vi "强度图.vi"() -> ()   [LabVIEW 2020]
doc: "本VI是为《我和LabVIEW》一书编写的示例。\n关于本书的介绍请参考网页：\nhttp://ruanqizhen.spaces.live.com/blog/cns!5852D4F797C53FB6!4310.entry"
panel:
  out "表格控件":string[][](table)
  out "强度图":dbl[][](graph)
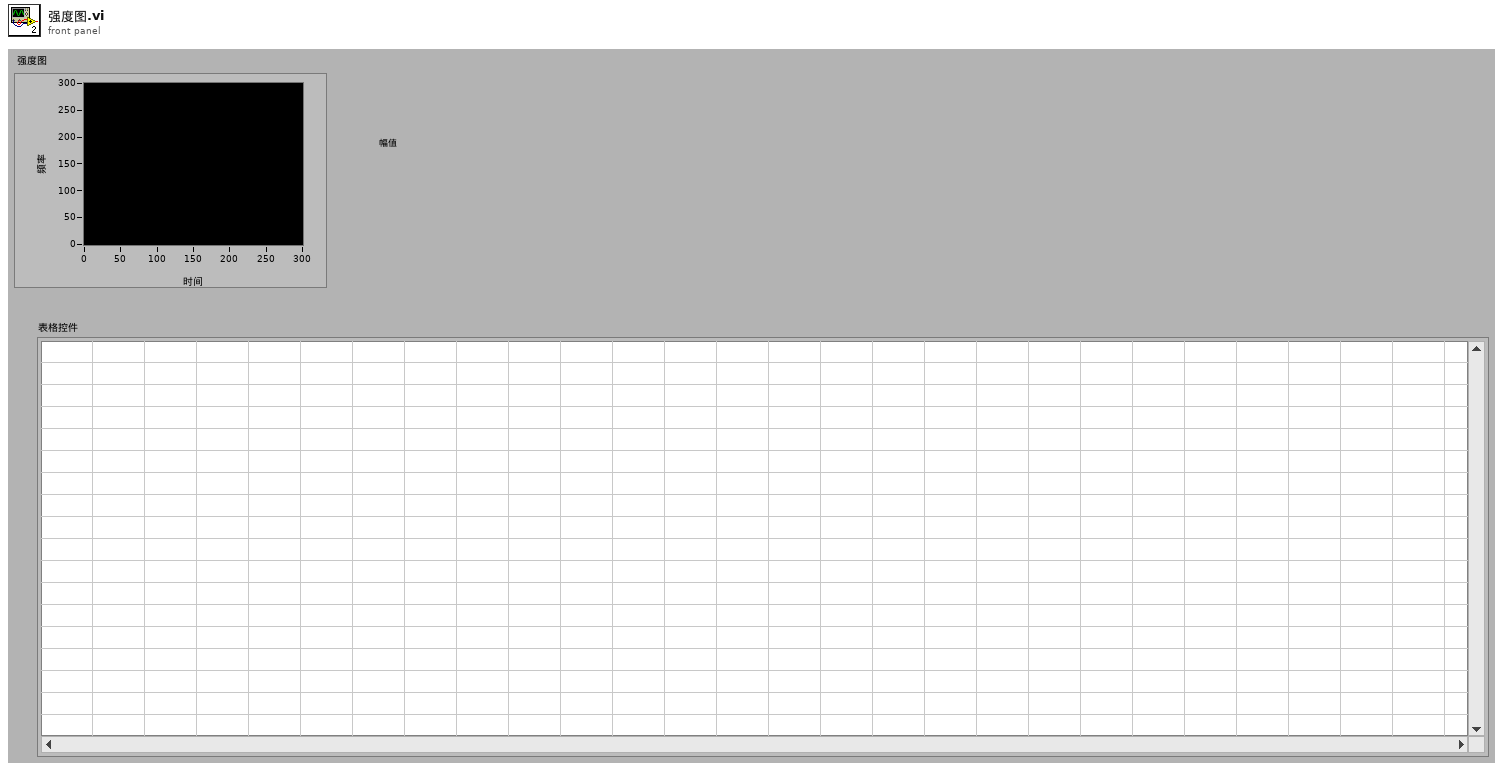
[diagram p1: front panel]
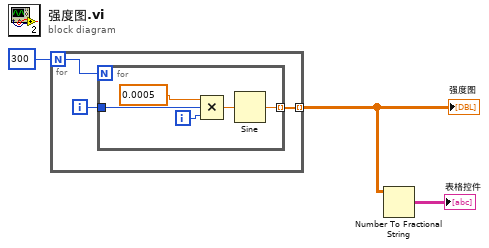
[diagram p0: block diagram]
diagram:
  n1 = for {
    N: 300 -> [w5]
    tunnel: [w4] -> w2 mode=indexing
    i -> [w6]
    n2 = for {
      N: w5 -> [_]
      tunnel: w6 -> [w10]
      tunnel: [w7] -> w4 mode=indexing
      i -> [w9]
      n3 = Compound Arithmetic op=MULTIPLY(0.0005 ("y"), w10, w9) -> (w8:dbl)
      n4 = Sine(x=w8) -> (sin(x)=w7:dbl)
    }
  }
  "强度图" <- w2
  n5 = Number To Fractional String(number=w2) -> (F-format string=→"表格控件":string[][])  [unwired: 3 out]
